vi "norm 3D array.vi"(3 "Vector":dbl[][](array[numeric]) format="%.2f") -> (0 "|x|":dbl[](array[numeric]) format="%.2f", 1 "x/|x|":dbl[][](array[numeric]) format="%.2f")   [LabVIEW 2016, in "impulse functions.lvlib"]
uses:
  impulse functions.lvlib
panel:
  # "Copyright Americo A. Migliaccio (c) 2002 All Rights Reserved by Author"
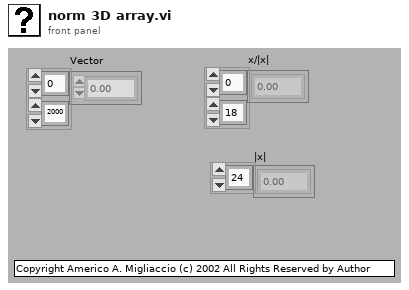
[diagram p1: front panel]
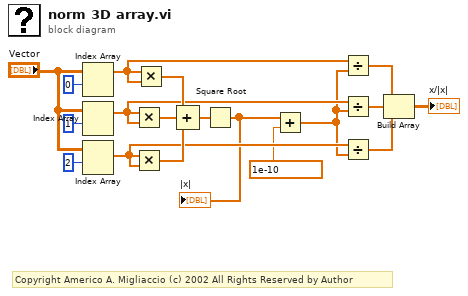
[diagram p0: block diagram]
diagram:
  # "Copyright Americo A. Migliaccio (c) 2002 All Rights Reserved by Author"
  n1 = Index Array(array="Vector", index (row)=0 ("Index (row)")) -> (element=w11:dbl[])  [unwired: 1 in]
  n2 = Index Array(array="Vector", index (row)=1 ("Index (row)")) -> (element=w10:dbl[])  [unwired: 1 in]
  n3 = Index Array(array="Vector", index (row)=2 ("Index (row)")) -> (element=w9:dbl[])  [unwired: 1 in]
  n4 = Multiply(x=w10, y=w10) -> (x*y=w13:dbl[])
  n5 = Multiply(x=w9, y=w9) -> (x*y=w12:dbl[])
  n6 = Multiply(x=w11, y=w11) -> (x*y=w14:dbl[])
  n7 = Compound Arithmetic op=ADD(w14, w13, w12) -> (w8:dbl[])
  n8 = Square Root(x=w8) -> (sqrt(x)=w3:dbl[])
  "|x|" <- w3
  n9 = Add(x=w3, y=1e-10 ("Index (row)")) -> (x+y=w2:dbl[])
  n10 = Divide(x=w11, y=w2) -> (x/y=w7:dbl[])
  n11 = Divide(x=w10, y=w2) -> (x/y=w6:dbl[])
  n12 = Divide(x=w9, y=w2) -> (x/y=w5:dbl[])
  n13 = Build Array(w7, w6, w5) -> (→"x/|x|":dbl[][])
